vi "Differential_Drive_Kinematics_Curvature_Control.vi"(8 "Scale_Down_For_Turn":bool, 9 "Angular_Throttle":dbl, 10 "Linear_Throttle":dbl) -> (1 "Right_Motor_Velocity(rotations/s)":dbl, 2 "Left_Motor_Velocity(rotations/s)":dbl)   [LabVIEW 2019]
panel:
  in  "turn_in_place_limit":dbl=0.01
  in  "max_curvature(1/in)(aka 1/min_radius)":dbl=0.06667
  in  "Gear_Reduction(output/input)":dbl=1.0
  in  "Wheel_Base_Radius(in)":dbl=11.87
  in  "Wheel_Radius(in)":dbl=3.0
  in  "Max_Angular_Speed(rad/s)":dbl=7.5
  in  "Max_Linear_Speed(in/s)":dbl=170.0
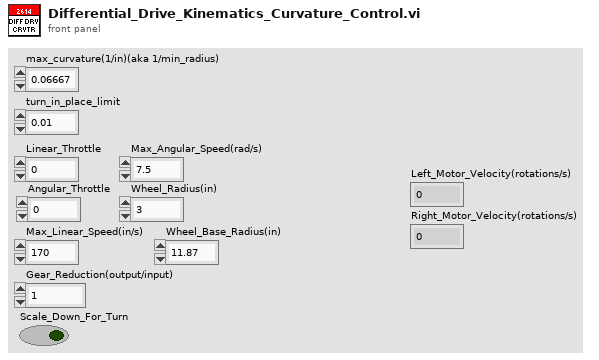
[diagram p1: front panel]
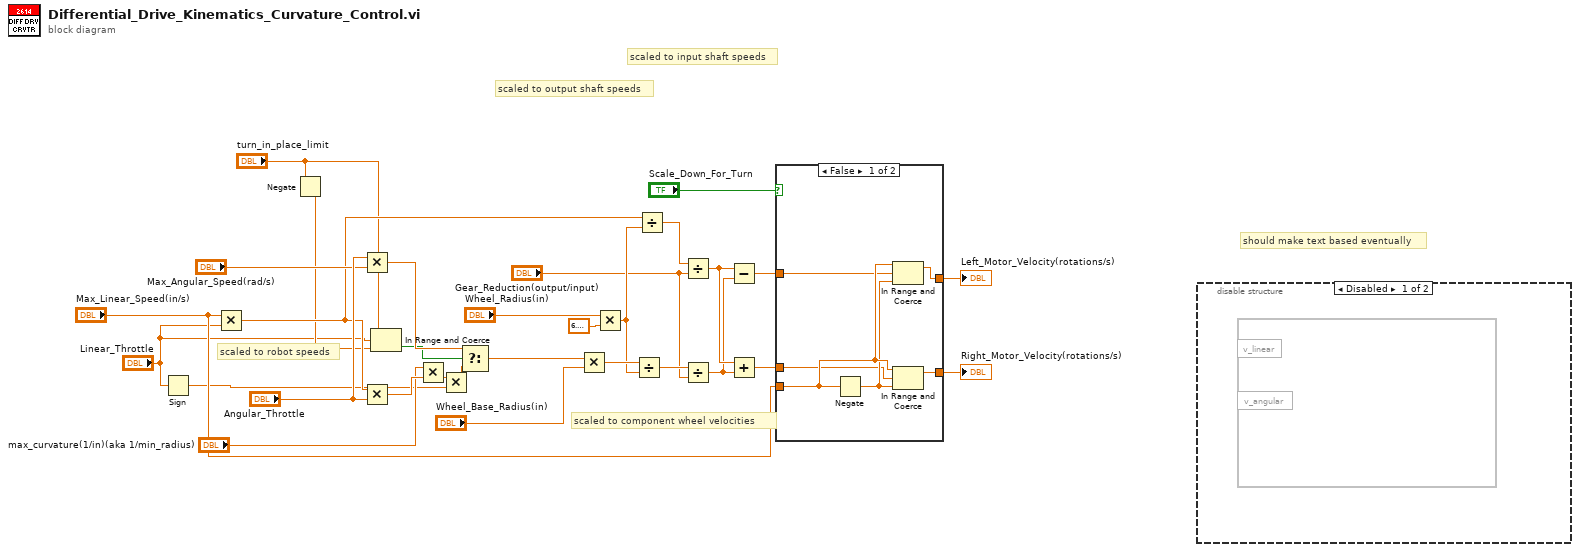
[diagram p0: block diagram]
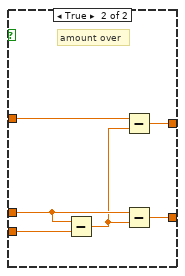
[diagram p3: hidden frame]
diagram:
  # "should make text based eventually"
  # "scaled to component wheel velocities"
  # "scaled to input shaft speeds"
  # "scaled to output shaft speeds"
  # "scaled to robot speeds"
  n1 = Sign(1:"Linear_Throttle") -> (0:w1:dbl)
  n2 = Multiply(x="Max_Linear_Speed(in/s)", y="Linear_Throttle") -> (x*y=w7:dbl)
  n3 = Negate(x="turn_in_place_limit") -> (-x=w5:dbl)
  n4 = Multiply(x="Angular_Throttle", y="Max_Angular_Speed(rad/s)") -> (x*y=w9:dbl)
  n5 = Multiply(x=w7, y="Angular_Throttle") -> (x*y=w14:dbl)
  n6 = In Range and Coerce(upper limit="turn_in_place_limit", x="Linear_Throttle", lower limit=w5) -> (In Range?=w8:bool)  [unwired: 1 out]
  n7 = Multiply(x="max_curvature(1/in)(aka 1/min_radius)", y=w14) -> (x*y=w2:dbl)
  n8 = Multiply(x=w2, y=w1) -> (x*y=w3:dbl)
  n9 = Select(t=w9, s=w8, f=w3) -> (s? t:f=w12:dbl)
  n10 = Multiply(x=w12, y="Wheel_Base_Radius(in)") -> (x*y=w26:dbl)
  n11 = Multiply(x="Wheel_Radius(in)", y=6.283185307179586) -> (x*y=w25:dbl)
  n12 = Divide(x=w26, y=w25) -> (x/y=w24:dbl)
  n13 = Divide(x=w7, y=w25) -> (x/y=w28:dbl)
  n14 = Divide(x=w28, y="Gear_Reduction(output/input)") -> (x/y=w22:dbl)
  n15 = Divide(x=w24, y="Gear_Reduction(output/input)") -> (x/y=w21:dbl)
  n16 = Subtract(x=w22, y=w21) -> (x-y=w18:dbl)
  n17 = Add(x=w22, y=w21) -> (x+y=w17:dbl)
  n18 = case shown="False" "Scale_Down_For_Turn" {
    tunnel: "Max_Linear_Speed(in/s)" -> [w36 w42]
    tunnel: w18 -> [w34 w39]
    tunnel: w17 -> [w33 w40]
    tunnel: [w32 w41] -> w16
    tunnel: [w31 w37] -> w15
    frame False {
      n19 = Negate(x=w36) -> (-x=w35:dbl)
      n20 = In Range and Coerce(upper limit=w36, x=w34, lower limit=w35) -> (coerced(x)=w31:dbl)  [unwired: 1 out]
      n21 = In Range and Coerce(upper limit=w36, x=w33, lower limit=w35) -> (coerced(x)=w32:dbl)  [unwired: 1 out]
    }
    frame True {
      # "amount over"
      n22 = Subtract(x=w40, y=w42) -> (x-y=w38:dbl)
      n23 = Subtract(x=w39, y=w38) -> (x-y=w37:dbl)
      n24 = Subtract(x=w40, y=w38) -> (x-y=w41:dbl)
    }
  }
  "Right_Motor_Velocity(rotations/s)" <- w16
  "Left_Motor_Velocity(rotations/s)" <- w15
  n25 = disable-structure shown="Disabled" {
    frame Disabled {
      n26 = formula code=""() -> ()  [unwired: 2 in]
    }
    frame Enabled {
    }
  }
